vi "Write (no data).vi"(8 "error in (no error)":errorcluster, 10 "Label":string) -> (0 "error out":errorcluster, 3 "Message":refnum<class "MSG.lvclass">)   [LabVIEW 2011, in "Messenging.lvlib" / "MSG.lvclass"]
uses:
  MSG.lvclass
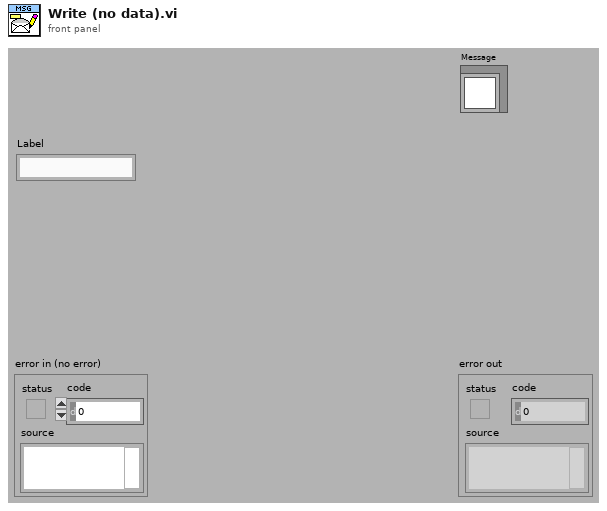
[diagram p1: front panel]
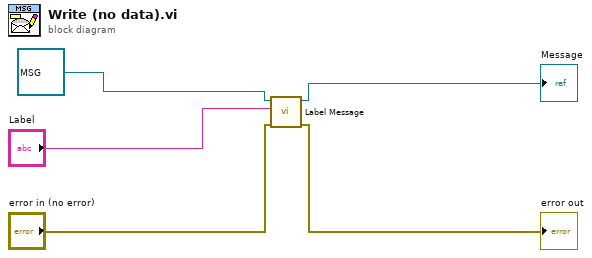
[diagram p0: block diagram]
diagram:
  n1 = call-dynamic "Label Message.vi"("error in (no error)"="error in (no error)", "Label"="Label", "Message"=refnum<class "MSG.lvclass"> refnum ("Message.lvclass in")) -> ("error out"=→"error out":errorcluster, "Message"=→"Message":refnum<class "MSG.lvclass">)  [unwired: 7 out]
